vi "Build Tree Items.vi"(8 "error in (no error)":errorcluster, 10 "Item Indent":i32, 11 "Variant":variant) -> (0 "error out":errorcluster, 3 "Items out":T1(array[cluster]))   [LabVIEW 2017, in "Variant Tree API.lvlib"]
uses:
  Variant Tree API.lvlib
  <vilib>/National Instruments/Variant JSON API/Variant JSON API.lvlib
  <vilib>/National Instruments/Variant Data Manipulation/Variant Data Manipulation.lvlib
  <vilib>/Utility/Data Type/NI_Data Type.lvlib
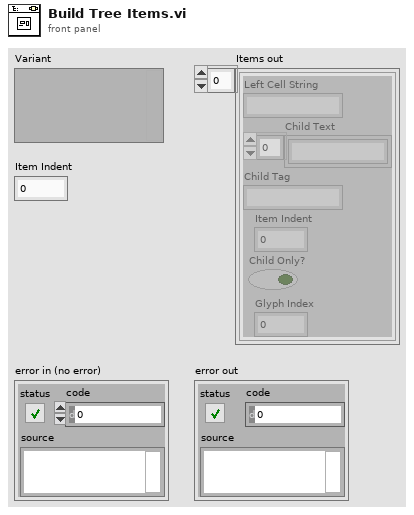
[diagram p1: front panel]
types:
  T1 = cluster{"Left Cell String":string, "Child Text":string[], "Child Tag":string, "Item Indent":i32, "Child Only?":bool, "Glyph Index":i32}[]
  T2 = typedef "NI_Data Type.lvlib/Data Type.ctl" = enum8{"Invalid Type", "Void", "I8", "I16", "I32", "I64", "U8", "U16", "U32", "U64", "Single Float", "Double Float", "Extended Float", "Single Complex", "Double Complex", "Extended Complex", "Enum U8", "Enum U16", "Enum U32", "Enum U64", "Single Float With Unit", "Double Float With Unit", "Extended Float With Unit", "Single Complex with Unit", "Double Complex with Unit", "Extended Complex with Unit", "Boolean", "String", "Path", "Picture", "Tag", "Array", "Cluster", "Variant", "LV Variant", "Waveform", "Timestamp", "Digital Waveform", "Digital Data", "ExpressData", "Refnum", "External Data", "VI", "Poly VI", "LabVIEW Class Instance", "Fixed Point"}
  T3 = cluster{"Left Cell String":string, "Child Text":string[], "Child Tag":string, "Item Indent":i32, "Child Only?":bool, "Glyph Index":i32}
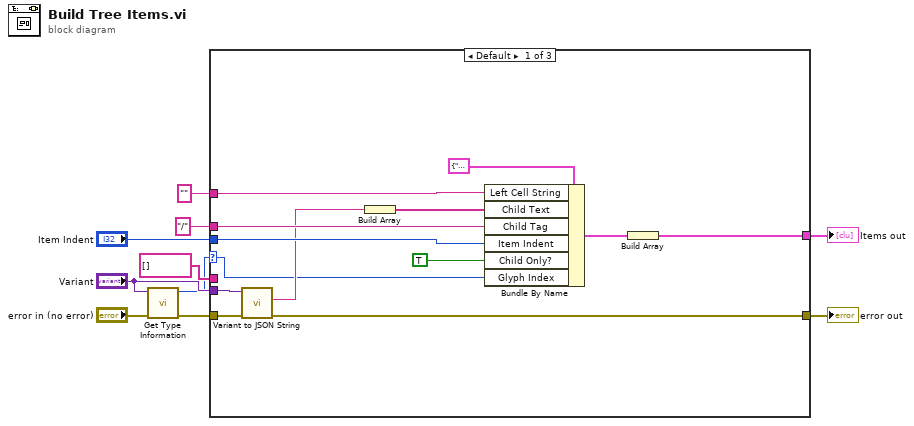
[diagram p0: block diagram]
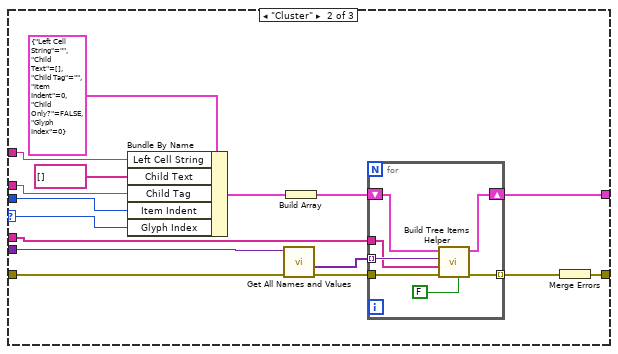
[diagram p2: hidden frame]
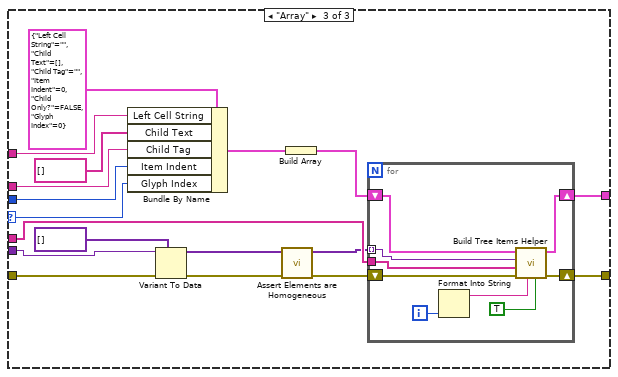
[diagram p3: hidden frame]
diagram:
  n1 = call <vilib>:"Get Type Information.vi"("error in (no error)"="error in (no error)", "Variant"="Variant") -> ("error out"=w3:errorcluster, "Type"=w1:T2)  [unwired: 5 in, 3 out]
  n2 = case shown="Default" w1 {
    selector: w1 -> [w11 w26 w51]
    tunnel: w3 -> [w16 w25 w61]
    tunnel: [w15 w36 w64] -> w6
    tunnel: "Variant" -> [w17 w39 w62]
    tunnel: [w20 w30 w60] -> w5
    tunnel: "" ("Name") -> [w12 w29 w56]
    tunnel: "Item Indent" -> [w19 w31 w54]
    tunnel: "/" ("path") -> [w18 w32 w55]
    tunnel: string[] [] ("Array in") -> [_ w28 w53]
    frame Default {
      n3 = call <vilib>:"Variant to JSON String.vi"("error in (no error)"=w16, "Variant in"=w17) -> ("error out"=w15:errorcluster, "String"=w14:string)  [unwired: 7 in, 1 out]
      n4 = Build Array(w14) -> (w13:string[])
      n5 = Bundle By Name(cluster=T3 {"Left Cell String"="", "Child Text"=[], "Child Tag"="", "Item Indent"=0, "Child Only?"=FALSE, "Glyph Index"=0} ("element"), "Left Cell String"=w12, "Child Text"=w13, "Child Tag"=w18, "Item Indent"=w19, "Child Only?"=TRUE, "Glyph Index"=w11) -> (w22:T3)
      n6 = Build Array(w22) -> (w20:T1)
    }
    frame "Cluster" {
      n7 = Bundle By Name(cluster=T3 {"Left Cell String"="", "Child Text"=[], "Child Tag"="", "Item Indent"=0, "Child Only?"=FALSE, "Glyph Index"=0} ("Items"), "Left Cell String"=w29, "Child Text"=string[] [], "Child Tag"=w32, "Item Indent"=w31, "Glyph Index"=w26) -> (w33:T3)
      n8 = call <vilib>:"Get All Names and Values.vi"("error in"=w25, "Cluster in"=w39) -> ("error out"=w24:errorcluster, "Values"=w38:variant[])  [unwired: 5 in, 3 out]
      n9 = Build Array(w33) -> (w34:T1)
      n10 = for {
        tunnel: w38 -> [w46] mode=indexing
        tunnel: [w45] -> w37 mode=indexing
        shift-right: [w42] -> w30
        shift-left: w34 -> [w43]
        tunnel: w24 -> [w41]
        tunnel: w28 -> [w40]
        n11 = call "Build Tree Items Helper.vi"("is array element?"=FALSE ("first call?"), "error in (no error)"=w41, "parents"=w40, "Variant"=w46, "Items"=w43) -> ("error out"=w45:errorcluster, "Items out"=w42:T1)  [unwired: 5 in]
      }
      n12 = Merge Errors(w37) -> (w36:errorcluster)
    }
    frame "Array" {
      n13 = Bundle By Name(cluster=T3 {"Left Cell String"="", "Child Text"=[], "Child Tag"="", "Item Indent"=0, "Child Only?"=FALSE, "Glyph Index"=0} ("Items"), "Left Cell String"=w56, "Child Text"=string[] [], "Child Tag"=w55, "Item Indent"=w54, "Glyph Index"=w51) -> (w58:T3)
      n14 = Variant To Data(error in=w61, type=variant[] [], Variant=w62) -> (data=w50:variant[], error out=w48:errorcluster)
      n15 = call <vilib>:"Assert Elements are Homogeneous.vi"("error in (no error)"=w48, "array in"=w50) -> ("error out"=w47:errorcluster, "array out"=w49:variant[])  [unwired: 8 in]
      n16 = Build Array(w58) -> (w57:T1)
      n17 = for {
        tunnel: w49 -> [w70] mode=indexing
        shift-right: [w73] -> w64
        shift-left: w47 -> [w72]
        shift-right: [w68] -> w60
        shift-left: w57 -> [w69]
        tunnel: w53 -> [w65]
        i -> [w67]
        n18 = Format Into String(w67) -> (resulting string=w66:string)  [unwired: 3 in, 1 out]
        n19 = call "Build Tree Items Helper.vi"("is array element?"=TRUE ("first call?"), "index string"=w66, "error in (no error)"=w72, "parents"=w65, "Variant"=w70, "Items"=w69) -> ("error out"=w73:errorcluster, "Items out"=w68:T1)  [unwired: 4 in]
      }
    }
  }
  "error out" <- w6
  "Items out" <- w5
